vi "String NotContain.vi"(11 "Data In":string) -> (3 "Data Out":string)   [LabVIEW 2018]
uses:
  Core/Assert API Components/Failure Actions.ctl
  Core/Assert API Components/Assert API Components.lvlib
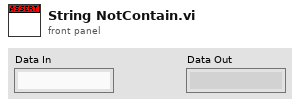
[diagram p1: front panel]
types:
  T1 = typedef "Assert API Components.lvlib/Failure Actions.ctl" = enum16{"None", "Log To File", "Pause Execution", "Abort Execution"}
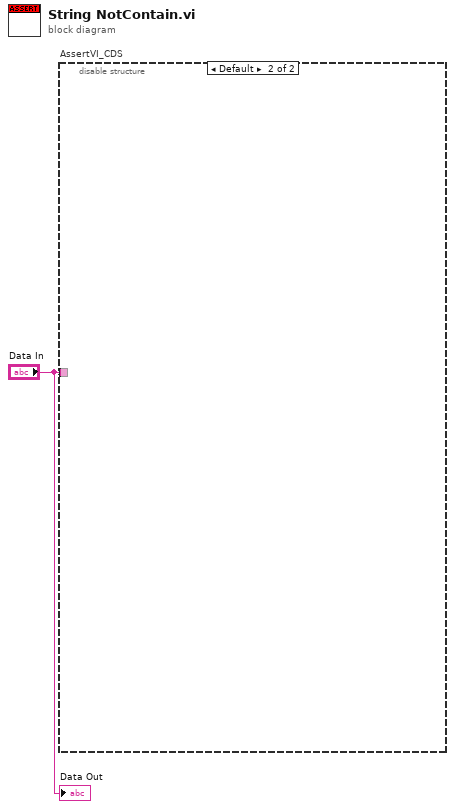
[diagram p0: block diagram]
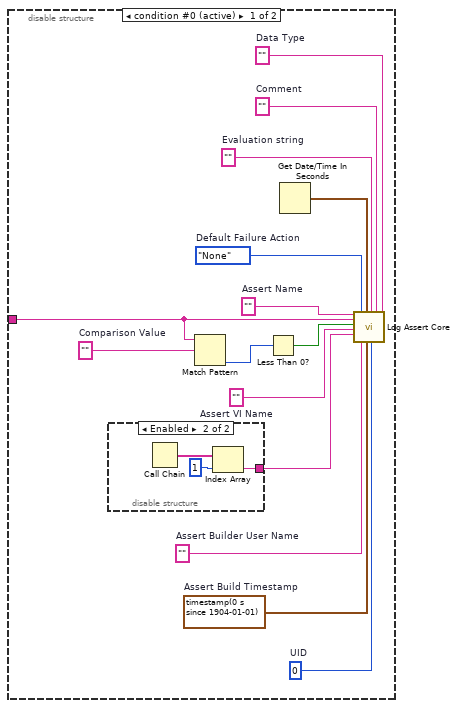
[diagram p2: hidden frame]
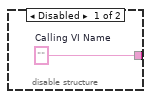
[diagram p3: hidden frame]
diagram:
  n1 = disable-structure "AssertVI_CDS" shown="Default" {
    disable-tunnel: "Data In" -> [w12 _]
    frame condition #0 (active) {
      w3 = 0  # UID
      w5 = ""  # Assert VI Name
      w6 = ""  # Assert Builder User Name
      w7 = timestamp(0 s since 1904-01-01)  # Assert Build Timestamp
      w8 = ""  # Data Type
      w14 = ""  # Comment
      w13 = ""  # Evaluation string
      w15 = Failure_Actions."None"  # Default Failure Action
      w16 = ""  # Assert Name
      w11 = ""  # Comparison Value
      n2 = disable-structure shown="Enabled" {
        disable-tunnel: [w17 w18] -> w2
        frame Disabled {
          w17 = ""  # Calling VI Name
        }
        frame Enabled {
          n3 = Call Chain() -> (call chain=w19:string[])
          n4 = Index Array(array=w19, index=1) -> (element=w18:string)
        }
      }
      n5 = Match Pattern(string=w12, regular expression=w11) -> (offset past match=w10:i32)  [unwired: 1 in, 3 out]
      n6 = Less Than 0?(x=w10) -> (x < 0?=w9:bool)
      n7 = Get Date/Time In Seconds() -> (seconds since 1Jan1904=w4:timestamp)
      n8 = call "Log Assert Core.vi"("Assert Name"=w16, "Data Value"=w12, "Status"=w9, "Assert VI Name"=w5, "Calling VI Name"=w2, "Failure Action"=w15, "Assert Builder User Name"=w6, "Last Update"=w4, "Assert Build Timestamp"=w7, "Evaluation String"=w13, "Assert VI UID"=w3, "Comment"=w14, "Data Type"=w8) -> ()  [unwired: 7 in]
    }
    frame condition #1 {
    }
  }
  "Data Out" <- "Data In"
